vi "Cleanup.vi"(8 "error in (no error)":errorcluster, 11 "Timer Demo App in":refnum<class "Timer Demo App.lvclass">) -> (0 "error out":errorcluster)   [LabVIEW 2020, in "Timer Demo.lvlib" / "Timer Demo App.lvclass"]
uses:
  Timer Demo App.lvclass
  lv-http-server/HTTP Server/Server/Server.lvclass
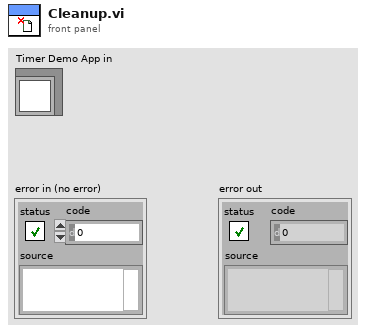
[diagram p1: front panel]
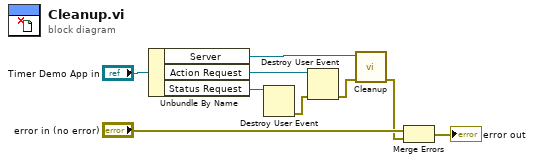
[diagram p0: block diagram]
diagram:
  n1 = Unbundle By Name("Timer Demo App in") -> ("Server"=w5:refnum<class "Server.lvclass">, "Action Request"=w6:refnum<user-event>, "Status Request"=w7:refnum<user-event>)
  n2 = Destroy User Event(user event=w7) -> (error out=w3:errorcluster)  [unwired: 1 in]
  n3 = Destroy User Event(user event=w6, error in=w3) -> (error out=w4:errorcluster)
  n4 = call "Cleanup.vi"("error in (no error)"=w4, "Server in"=w5) -> ("error out"=w1:errorcluster)  [unwired: 9 in]
  n5 = Merge Errors("error in (no error)", w1) -> (→"error out":errorcluster)
